vi "Menu.Sequence.Load.vi"(8 "error in (no error)":errorcluster, 9 "MenuRef":refnum<k9>, 10 "Coords":T1, 11 "Cluster in":T2) -> (0 "error out":errorcluster, 3 "Cluster out":T2)   [LabVIEW 2013, in "Simple Sequence Editor.lvlib"]
uses:
  Simple Sequence Editor.lvlib
  Types/StateVariables.ctl
  Types/ChannelProperties.ctl
  <vilib>/Utility/miscctls.llb/LVPoint32TypeDef.ctl
  Constants.vi
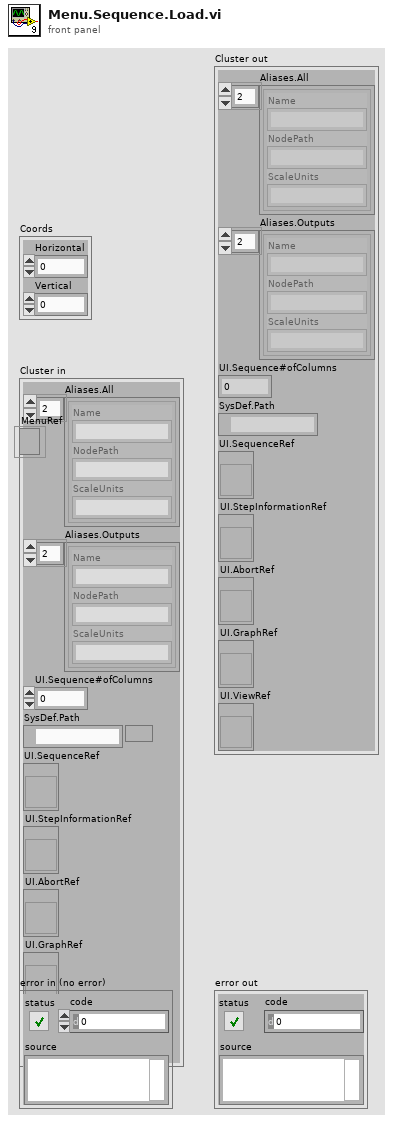
[diagram p1: front panel]
types:
  T1 = typedef "LVPoint32TypeDef.ctl" = cluster{"Horizontal":i32, "Vertical":i32}
  T2 = typedef "Simple Sequence Editor.lvlib/StateVariables.ctl" = cluster{"Aliases.All":T3[], "Aliases.Outputs":T3[], "UI.Sequence#ofColumns":i32, "SysDef.Path":path, "UI.SequenceRef":refnum<vi>, "UI.StepInformationRef":refnum<vi>, "UI.AbortRef":refnum<vi>, "UI.GraphRef":refnum<vi>, "UI.ViewRef":refnum<vi>}
  T3 = typedef "Simple Sequence Editor.lvlib/ChannelProperties.ctl" = cluster{"Name":string, "NodePath":string, "ScaleUnits":string}
  T4 = typedef "LVRowAndColumnTypeDef.ctl" = cluster{"Row":i32, "Column":i32}
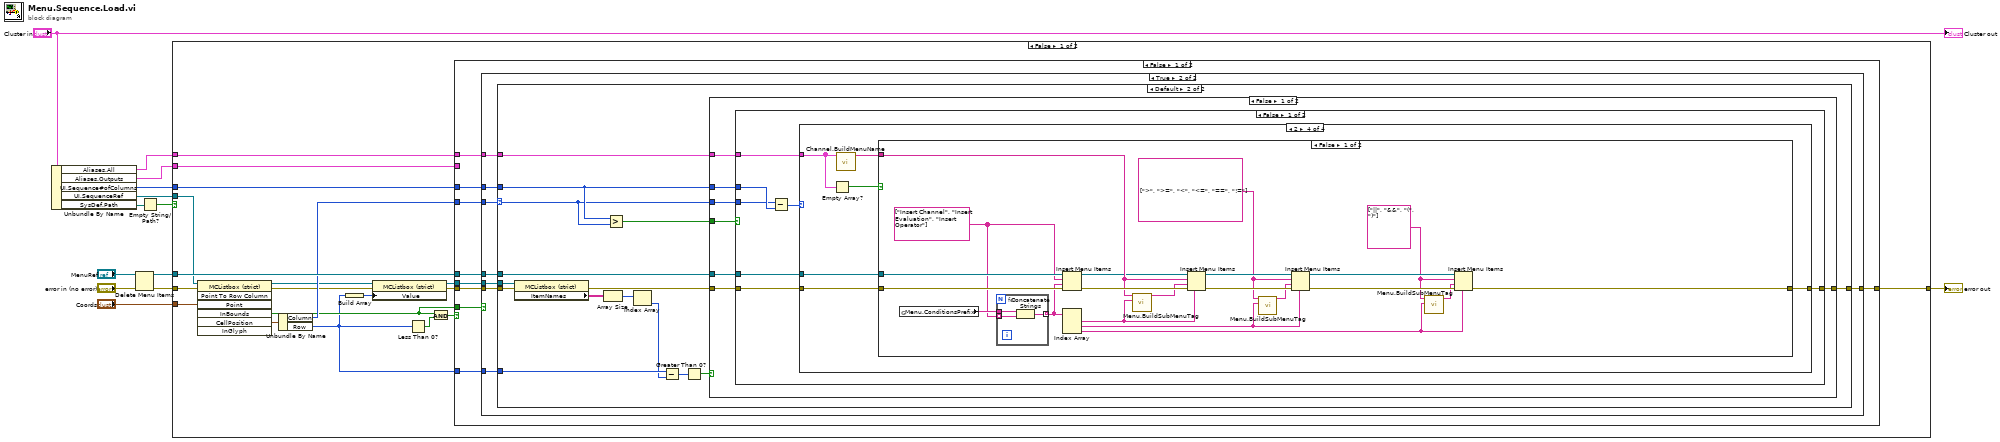
[diagram p0: block diagram]
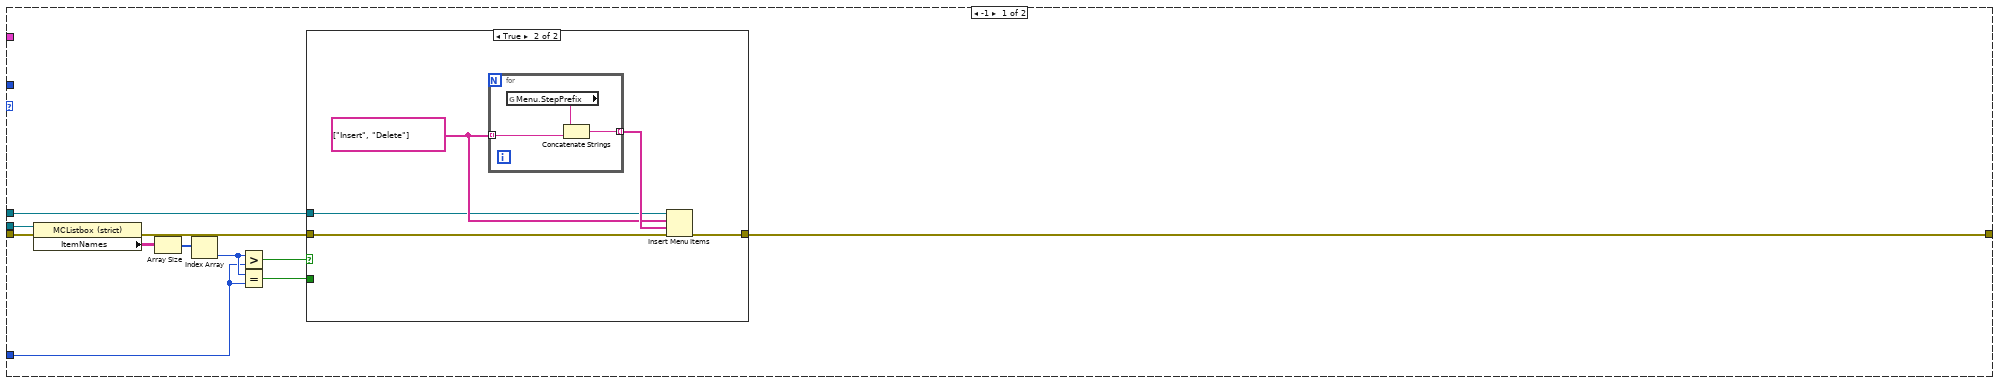
[diagram p3: hidden frame]
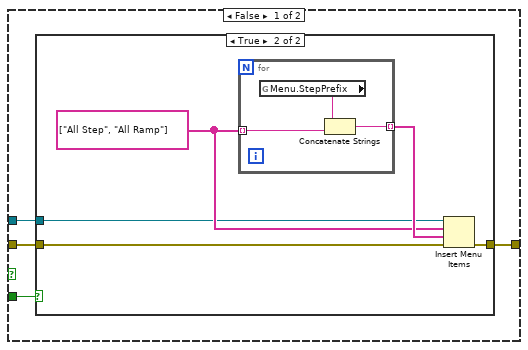
[diagram p4: hidden frame]
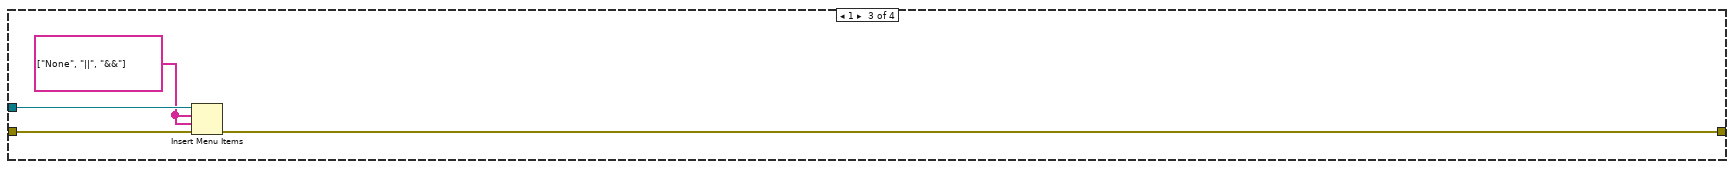
[diagram p8: hidden frame]
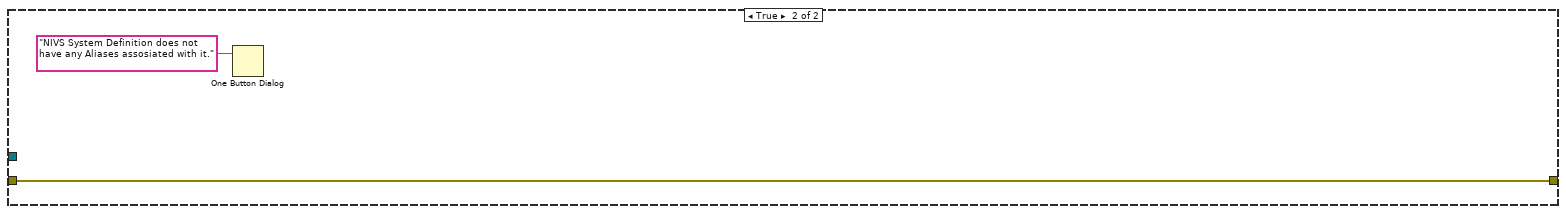
[diagram p9: hidden frame]
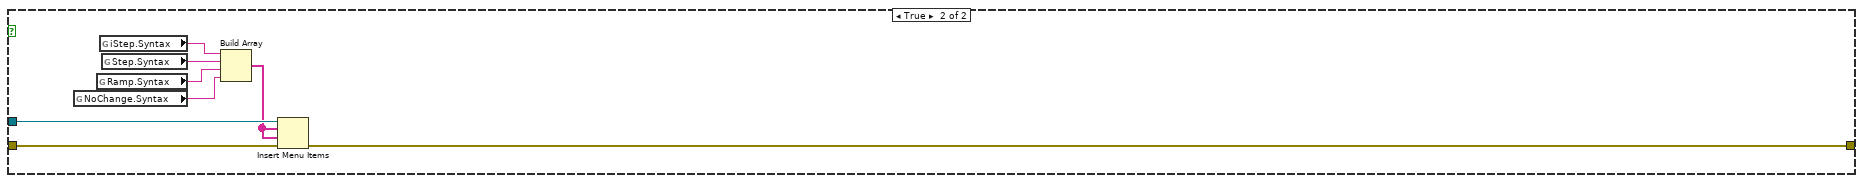
[diagram p10: hidden frame]
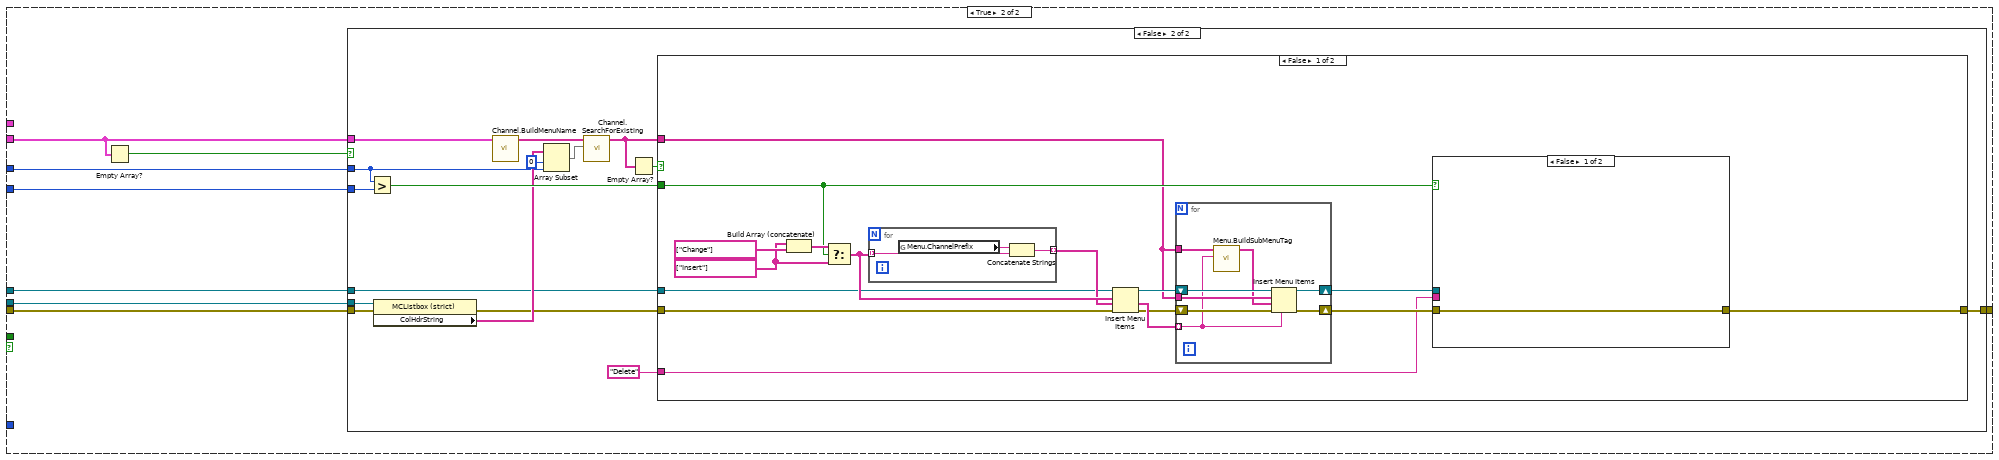
[diagram p12: hidden frame]
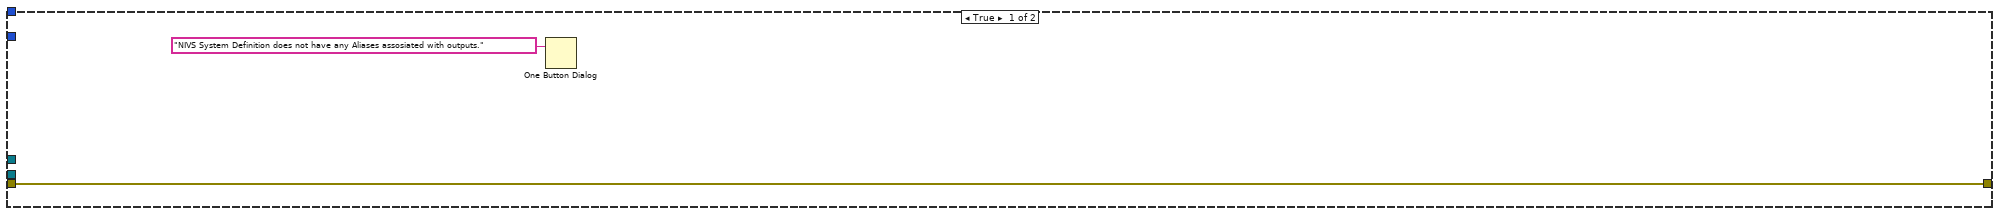
[diagram p13: hidden frame]
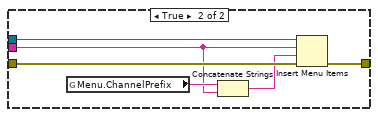
[diagram p14: hidden frame]
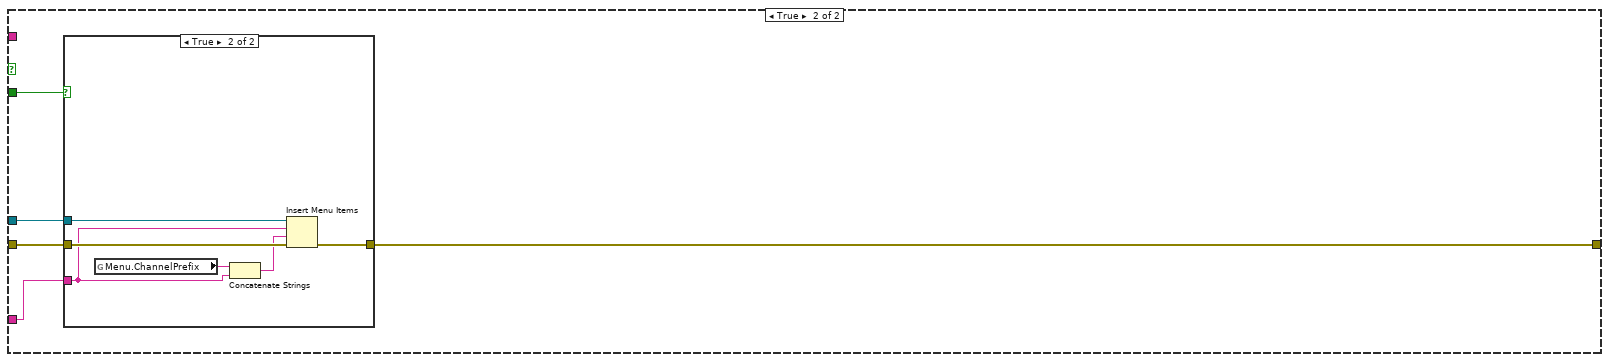
[diagram p15: hidden frame]
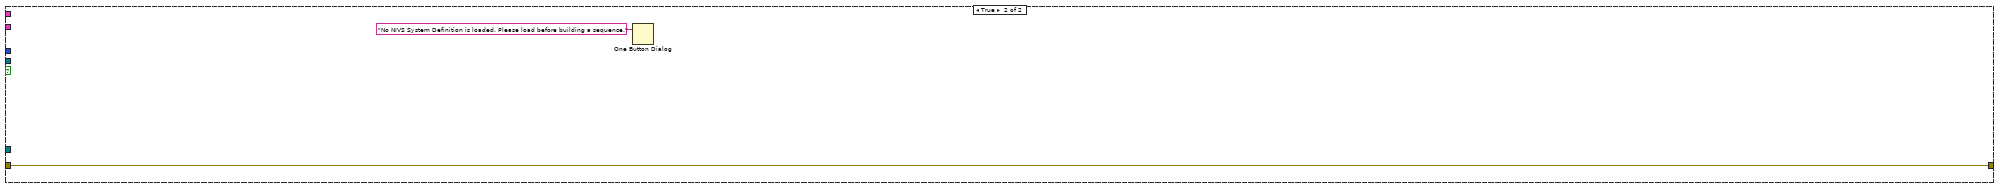
[diagram p17: hidden frame]
diagram:
  n1 = Unbundle By Name("Cluster in") -> ("Aliases.All"=w1:T3[], "Aliases.Outputs"=w9:T3[], "UI.Sequence#ofColumns"=w12:i32, "UI.SequenceRef"=w10:refnum<vi>, "SysDef.Path"=w7:path)
  n2 = Delete Menu Items(6:"error in (no error)", 9:"MenuRef") -> (0:w4:errorcluster, 3:w2:refnum<k9>)  [unwired: 2 in]
  n3 = Empty String/Path?(string/path=w7) -> (empty?=w6:bool)
  n4 = case shown="False" w6 {
    tunnel: [w32 w231] -> w13
    tunnel: w2 -> [w31 _]
    tunnel: w12 -> [w30 _]
    tunnel: "Coords" -> [w25 _]
    tunnel: w10 -> [w24 _]
    tunnel: w4 -> [w23 w231]
    tunnel: w9 -> [w22 _]
    tunnel: w1 -> [w20 _]
    frame False {
      n5 = invoke class="MCListbox (strict)" method="Point To Row Column"(reference=w24, error in=w23, "Point"=w25) -> (reference out=w18:refnum<vi>, error out=w19:errorcluster, "InBounds"=w21:bool, "CellPosition"=w26:T4)  [unwired: 4 in, 3 out]
      n6 = Unbundle By Name(w26) -> ("Column"=w29:i32, "Row"=w15:i32)
      n7 = Build Array(w15) -> (w14:i32[])
      n8 = property class="MCListbox (strict)"(reference=w18, error in=w19, "Value"=w14) -> (reference out=w16:refnum<vi>, error out=w17:errorcluster)
      n9 = Less Than 0?(x=w15) -> (x < 0?=w27:bool)
      n10 = And(x=w21, y=w27) -> (x .and. y?=w28:bool)
      n11 = case shown="False" w28 {
        tunnel: w29 -> [w36 w166]
        tunnel: w30 -> [w37 w164]
        tunnel: w31 -> [w35 w161]
        tunnel: w17 -> [w40 w162]
        tunnel: [w34 w163] -> w32
        tunnel: w16 -> [w39 w165]
        tunnel: w22 -> [_ w160]
        tunnel: w21 -> [w41 _]
        tunnel: w15 -> [w38 _]
        tunnel: w20 -> [w33 _]
        frame False {
          n12 = case shown="True" w41 {
            tunnel: w40 -> [w42 w49]
            tunnel: w39 -> [_ w50]
            tunnel: w38 -> [_ w48]
            tunnel: w37 -> [_ w47]
            tunnel: w36 -> [_ w46]
            tunnel: w35 -> [_ w45]
            tunnel: [w42 w44] -> w34
            tunnel: w33 -> [_ w43]
            frame False {
            }
            frame True {
              n13 = case shown="Default" w46 {
                selector: w46 -> [_ w87]
                tunnel: w50 -> [w57 w97]
                tunnel: w49 -> [w59 w96]
                tunnel: w48 -> [w52 w93]
                tunnel: w47 -> [_ w88]
                tunnel: w45 -> [w60 w89]
                tunnel: [w61 w85] -> w44
                tunnel: w43 -> [_ w83]
                frame -1 {
                  n14 = property class="MCListbox (strict)"(reference=w57, error in=w59) -> (error out=w58:errorcluster, "ItemNames"=w55:string[][])  [unwired: 1 out]
                  n15 = Array Size(array=w55) -> (size(s)=w56:i32[])
                  n16 = Index Array(array=w56) -> (element=w53:i32)  [unwired: 1 in]
                  n17 = Greater?(x=w53, y=w52) -> (0:w54:bool)
                  n18 = Equal?(x=w53, y=w52) -> (x = y?=w51:bool)
                  n19 = case shown="True" w54 {
                    tunnel: [w64 w79] -> w61
                    tunnel: w60 -> [w63 w76]
                    tunnel: w58 -> [w65 w75]
                    tunnel: w51 -> [w62 _]
                    frame False {
                      n20 = case shown="True" w62 {
                        tunnel: w65 -> [w66 w69]
                        tunnel: [w66 w68] -> w64
                        tunnel: w63 -> [_ w67]
                        frame False {
                        }
                        frame True {
                          w70 = string[] ["All Step", "All Ramp"] ("item names")
                          n21 = for {
                            tunnel: [w73] -> w71 mode=indexing
                            tunnel: w70 -> [w74] mode=indexing
                            n22 = global read "Constants.vi" "Menu.StepPrefix"() -> (w72:string)
                            n23 = Concatenate Strings(w72, w74) -> (w73:string)
                          }
                          n24 = Insert Menu Items(6:w69, 7:w71, 8:w70, 9:w67) -> (0:w68:errorcluster)  [unwired: 2 in, 2 out]
                        }
                      }
                    }
                    frame True {
                      w77 = string[] ["Insert", "Delete"] ("item names")
                      n25 = for {
                        tunnel: [w81] -> w78 mode=indexing
                        tunnel: w77 -> [w82] mode=indexing
                        n26 = global read "Constants.vi" "Menu.StepPrefix"() -> (w80:string)
                        n27 = Concatenate Strings(w80, w82) -> (w81:string)
                      }
                      n28 = Insert Menu Items(6:w75, 7:w78, 8:w77, 9:w76) -> (0:w79:errorcluster)  [unwired: 2 in, 2 out]
                    }
                  }
                }
                frame Default {
                  n29 = property class="MCListbox (strict)"(reference=w97, error in=w96) -> (error out=w91:errorcluster, "ItemNames"=w95:string[][])  [unwired: 1 out]
                  n30 = Array Size(array=w95) -> (size(s)=w94:i32[])
                  n31 = Greater?(x=w88, y=w87) -> (0:w86:bool)
                  n32 = Index Array(array=w94) -> (element=w92:i32)  [unwired: 1 in]
                  n33 = Subtract(x=w93, y=w92) -> (x-y=w84:i32)
                  n34 = Greater Than 0?(x=w84) -> (x > 0?=w90:bool)
                  n35 = case shown="False" w90 {
                    tunnel: w91 -> [w104 w158]
                    tunnel: w88 -> [w101 _]
                    tunnel: w87 -> [w100 _]
                    tunnel: w89 -> [w103 _]
                    tunnel: w86 -> [w102 _]
                    tunnel: [w99 w158] -> w85
                    tunnel: w83 -> [w98 _]
                    frame False {
                      n36 = case shown="False" w102 {
                        tunnel: w104 -> [w107 w157]
                        tunnel: w103 -> [w108 w155]
                        tunnel: w101 -> [w111 _]
                        tunnel: w100 -> [w110 _]
                        tunnel: [w106 w156] -> w99
                        tunnel: w98 -> [w105 _]
                        frame False {
                          n37 = Subtract(x=w110, y=w111) -> (x-y=w109:i32)
                          n38 = case shown="2" w109 {
                            tunnel: w108 -> [_ _ w117 w123]
                            tunnel: w107 -> [w112 w113 w116 w122]
                            tunnel: [w112 w113 w114 w121] -> w106
                            tunnel: w105 -> [_ _ _ w120]
                            frame Default {
                            }
                            frame 0 {
                            }
                            frame 1 {
                              w115 = string[] ["None", "||", "&&"] ("item names")
                              n39 = Insert Menu Items(6:w116, 7:w115, 8:w115, 9:w117) -> (0:w114:errorcluster)  [unwired: 2 in, 2 out]
                            }
                            frame 2 {
                              n40 = Empty Array?(array=w120) -> (empty?=w119:bool)
                              n41 = call "Channel.BuildMenuName.vi"("Aliases"=w120) -> ("Aliases Array"=w118:string[])  [unwired: 10 in]
                              n42 = case shown="False" w119 {
                                tunnel: w123 -> [w144 _]
                                tunnel: w122 -> [w143 w148]
                                tunnel: [w132 w148] -> w121
                                tunnel: w118 -> [w138 _]
                                frame False {
                                w125 = string[] [">", ">=", "<", "<=", "==", "!="] ("item names")
                                w124 = string[] ["||", "&&", "(", ")"] ("item names")
                                w141 = string[] ["Insert Channel", "Insert Evaluation", "Insert Operator"] ("item names")
                                n43 = global read "Constants.vi" "Menu.ConditionsPrefix"() -> (w142:string)
                                n44 = for {
                                tunnel: w141 -> [w147] mode=indexing
                                tunnel: w142 -> [w146]
                                tunnel: [w145] -> w135 mode=indexing
                                n45 = Concatenate Strings(w146, w147) -> (w145:string)
                                }
                                n46 = Insert Menu Items(6:w143, 7:w135, 8:w141, 9:w144) -> (0:w140:errorcluster, 3:w137:refnum<k9>)  [unwired: 2 in, 1 out]
                                n47 = Index Array(array=w135) -> (element #1=w136:string, element #2=w129:string, element #3=w127:string)  [unwired: 3 in]
                                n48 = call "Menu.BuildSubMenuTag.vi"("Menu"=w136, "Aliases Array"=w138) -> ("Tag Array"=w139:string[])  [unwired: 9 in]
                                n49 = Insert Menu Items(5:w136, 6:w140, 7:w139, 8:w138, 9:w137) -> (0:w134:errorcluster, 3:w131:refnum<k9>)  [unwired: 1 in, 1 out]
                                n50 = call "Menu.BuildSubMenuTag.vi"("Menu"=w129, "Aliases Array"=w125) -> ("Tag Array"=w128:string[])  [unwired: 9 in]
                                n51 = Insert Menu Items(5:w129, 6:w134, 7:w128, 8:w125, 9:w131) -> (0:w133:errorcluster, 3:w130:refnum<k9>)  [unwired: 1 in, 1 out]
                                n52 = call "Menu.BuildSubMenuTag.vi"("Menu"=w127, "Aliases Array"=w124) -> ("Tag Array"=w126:string[])  [unwired: 9 in]
                                n53 = Insert Menu Items(5:w127, 6:w133, 7:w126, 8:w124, 9:w130) -> (0:w132:errorcluster)  [unwired: 1 in, 2 out]
                                }
                                frame True {
                                n54 = One Button Dialog(message="NIVS System Definition does not have any Aliases assosiated with it.") -> ()  [unwired: 1 in, 1 out]
                                }
                              }
                            }
                          }
                        }
                        frame True {
                          n55 = global read "Constants.vi" "NoChange.Syntax"() -> (w151:string)
                          n56 = global read "Constants.vi" "Ramp.Syntax"() -> (w153:string)
                          n57 = global read "Constants.vi" "iStep.Syntax"() -> (w150:string)
                          n58 = global read "Constants.vi" "Step.Syntax"() -> (w154:string)
                          n59 = Build Array(w150, w154, w153, w151) -> (w152:string[])
                          n60 = Insert Menu Items(6:w157, 7:w152, 8:w152, 9:w155) -> (0:w156:errorcluster)  [unwired: 2 in, 2 out]
                        }
                      }
                    }
                    frame True {
                    }
                  }
                }
              }
            }
          }
        }
        frame True {
          n61 = Empty Array?(array=w160) -> (empty?=w159:bool)
          n62 = case shown="False" w159 {
            tunnel: w166 -> [_ w184]
            tunnel: w165 -> [_ w182]
            tunnel: w164 -> [_ w180]
            tunnel: [w168 w178] -> w163
            tunnel: w160 -> [_ w177]
            tunnel: w162 -> [w168 w173]
            tunnel: w161 -> [_ w174]
            frame True {
              n63 = One Button Dialog(message="NIVS System Definition does not have any Aliases assosiated with outputs.") -> ()  [unwired: 1 in, 1 out]
            }
            frame False {
              n64 = Greater?(x=w180, y=w184) -> (0:w183:bool)
              n65 = property class="MCListbox (strict)"(reference=w182, error in=w173) -> (error out=w172:errorcluster, "ColHdrString"=w181:string[])  [unwired: 1 out]
              n66 = call "Channel.BuildMenuName.vi"("Aliases"=w177) -> ("Aliases Array"=w175:string[])  [unwired: 10 in]
              n67 = Array Subset(array=w181, index=0, length=w180) -> (w176:string[])
              n68 = call "Channel.SearchForExisting.vi"("Existing Channels"=w176, "All Channels"=w175) -> ("Array out"=w171:string[])  [unwired: 9 in]
              n69 = Empty Array?(array=w171) -> (empty?=w170:bool)
              n70 = case shown="False" w170 {
                tunnel: w183 -> [w186 w219]
                tunnel: [w189 w222] -> w178
                tunnel: w174 -> [w193 w221]
                tunnel: w171 -> [w185 _]
                tunnel: w172 -> [w191 w223]
                tunnel: "Delete" ("string") -> [w187 w220]
                frame False {
                  w198 = string[] ["Insert"]
                  n71 = Build Array (concatenate)(w198, string[] ["Change"]) -> (w199:string[])
                  n72 = Select(t=w199, s=w186, f=w198) -> (s? t:f=w197:string[])
                  n73 = for {
                    tunnel: w197 -> [w218] mode=indexing
                    tunnel: [w217] -> w196 mode=indexing
                    n74 = global read "Constants.vi" "Menu.ChannelPrefix"() -> (w216:string)
                    n75 = Concatenate Strings(w216, w218) -> (w217:string)
                  }
                  n76 = Insert Menu Items(6:w191, 7:w196, 8:w197, 9:w193) -> (0:w192:errorcluster, 1:w194:string[], 3:w195:refnum<k9>)  [unwired: 2 in]
                  n77 = for {
                    tunnel: w194 -> [w210] mode=indexing
                    shift-right: [w214] -> w190
                    shift-left: w192 -> [w215]
                    tunnel: w185 -> [w212]
                    shift-right: [w211] -> w188
                    shift-left: w195 -> [w213]
                    tunnel: w185 -> [w209]
                    n78 = call "Menu.BuildSubMenuTag.vi"("Menu"=w210, "Aliases Array"=w209) -> ("Tag Array"=w208:string[])  [unwired: 9 in]
                    n79 = Insert Menu Items(5:w210, 6:w215, 7:w208, 8:w212, 9:w213) -> (0:w214:errorcluster, 3:w211:refnum<k9>)  [unwired: 1 in, 1 out]
                  }
                  n80 = case shown="False" w186 {
                    tunnel: w190 -> [w201 w207]
                    tunnel: [w201 w206] -> w189
                    tunnel: w188 -> [_ w205]
                    tunnel: w187 -> [_ w202]
                    frame False {
                    }
                    frame True {
                      n81 = global read "Constants.vi" "Menu.ChannelPrefix"() -> (w204:string)
                      n82 = Concatenate Strings(w204, w202) -> (w203:string)
                      n83 = Insert Menu Items(6:w207, 7:w203, 8:w202, 9:w205) -> (0:w206:errorcluster)  [unwired: 2 in, 2 out]
                    }
                  }
                }
                frame True {
                  n84 = case shown="True" w219 {
                    tunnel: w223 -> [w224 w230]
                    tunnel: [w224 w229] -> w222
                    tunnel: w221 -> [_ w228]
                    tunnel: w220 -> [_ w226]
                    frame False {
                    }
                    frame True {
                      n85 = global read "Constants.vi" "Menu.ChannelPrefix"() -> (w227:string)
                      n86 = Concatenate Strings(w227, w226) -> (w225:string)
                      n87 = Insert Menu Items(6:w230, 7:w225, 8:w226, 9:w228) -> (0:w229:errorcluster)  [unwired: 2 in, 2 out]
                    }
                  }
                }
              }
            }
          }
        }
      }
    }
    frame True {
      n88 = One Button Dialog(message="No NIVS System Definition is loaded. Please load before building a sequence.") -> ()  [unwired: 1 in, 1 out]
    }
  }
  "error out" <- w13
  "Cluster out" <- "Cluster in"
